vi "Panel.vi"(11 "ArrayHostPanel in":refnum<class "ArrayHostPanel.lvclass">) -> ()   [LabVIEW 2020, in "Nested.lvlib" / "ArrayHostPanel.lvclass"]
uses:
  ArrayHostPanel.lvclass
  C:/dev/lv/2020/lv-oopanel/OOPanel/Panel/Panel.lvclass
  OOPanel/Panel/Basic UI State.ctl
  ColorArrayPanel/ColorArrayPanel.lvclass
  C:/dev/lv/2020/lv-oopanel/OOPanel/ArrayPanel/ArrayPanel.lvclass
  OOPanel/ArrayManager/ArrayManager.lvclass
  OOPanel/Panel/Panel.lvclass
  OOPanel/OOPanel.lvlib
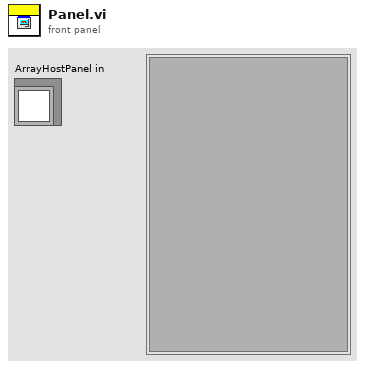
[diagram p1: front panel]
types:
  T1 = typedef "OOPanel.lvlib/Panel.lvclass/Basic UI State.ctl" = enum16{"Init", "Run", "Close"}
  T2 = typedef "OOPanel.lvlib/Panel.lvclass/Panel Events.ctl" = cluster{"Visbility":refnum<user-event>, "Close":refnum<user-event>}
  T3 = typedef "OOPanel.lvlib/Visibility State.ctl" = enum16{"Idle", "Closed", "Hidden", "Visible", "Subpanel", "Hidden Subpanel"}
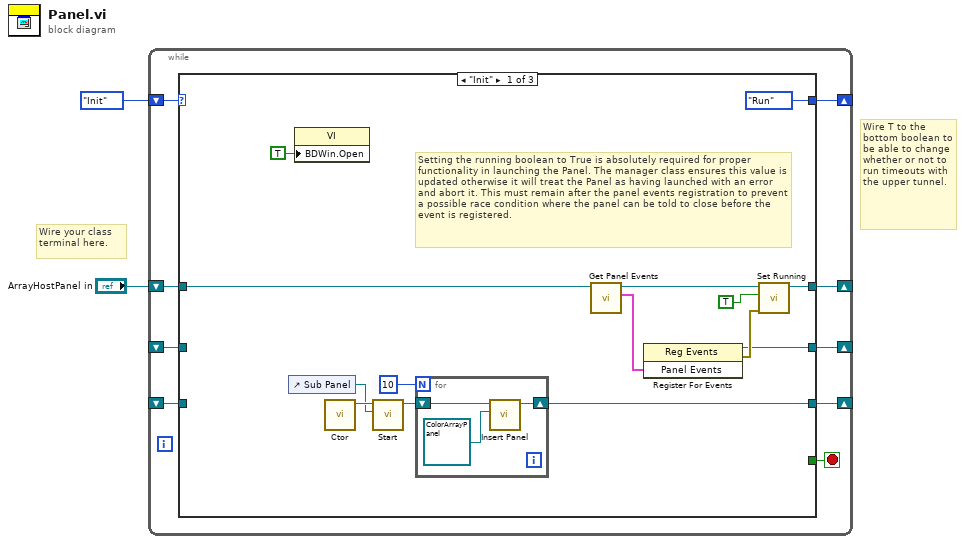
[diagram p0: block diagram]
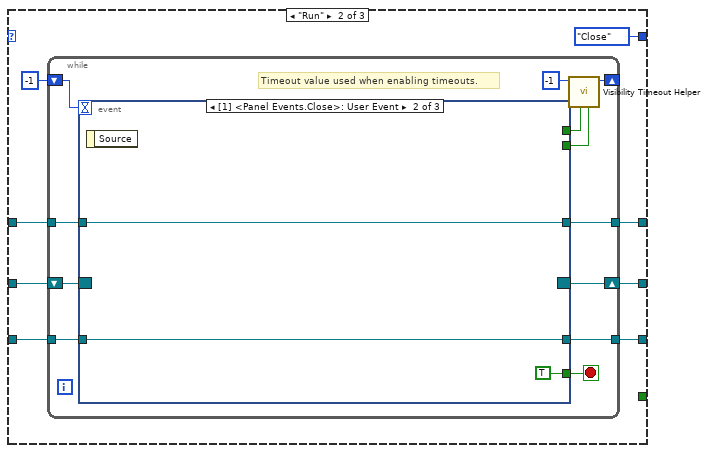
[diagram p2: hidden frame]
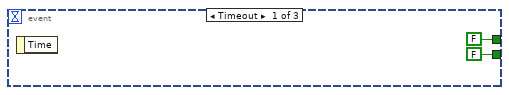
[diagram p3: hidden frame]
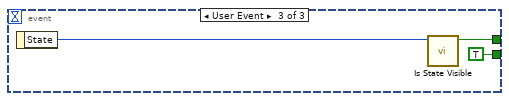
[diagram p4: hidden frame]
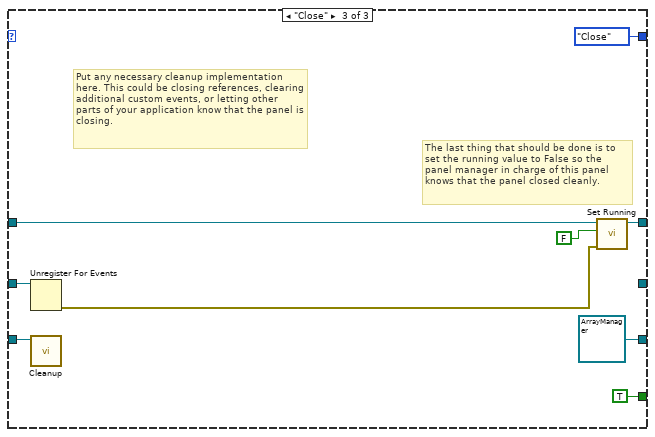
[diagram p5: hidden frame]
diagram:
  # "Wire T to the bottom boolean to be able to change whether or not to run timeouts with the upper tunnel."
  # "Wire your class terminal here."
  n1 = while {
    shift-right: [w10] -> _
    shift-left: _ -> [w11]
    shift-right: [w8] -> _
    shift-left: Basic_UI_State."Init" ("Basic UI State") -> [w9]
    shift-right: [w6] -> _
    shift-left: "ArrayHostPanel in" -> [w5]
    shift-right: [w4] -> _
    shift-left: _ -> [w3]
    stop <- w7 stop-if-true
    n2 = case shown="\"Init\"" w9 {
      tunnel: w11 -> [_ w36 w61]
      tunnel: [w22 w34 _] -> w10
      tunnel: [Basic_UI_State."Run" ("Basic UI State") Basic_UI_State."Close" ("Basic UI State") Basic_UI_State."Close" ("Basic UI State")] -> w8
      tunnel: [_ _ TRUE] -> w7
      tunnel: [w21 w31 w59] -> w6
      tunnel: w5 -> [w20 w32 w60]
      tunnel: [w13 w29 refnum<class "ArrayManager.lvclass"> refnum ("ArrayManager out")] -> w4
      tunnel: w3 -> [_ w30 w58]
      frame "Init" {
        # "Setting the running boolean to True is absolutely required for proper functionality in launching the Panel. The manager class ensures this value is updated otherwise it will treat the Panel as having launched with an error and abort it. This must remain after the panel events registration to prevent a possible race condition where the panel can be told to close before the event is registered."
        n3 = control-ref of="Sub Panel"() -> (w15:refnum<vi>)
        n4 = property class="VI"("BDWin.Open"=TRUE ("Block Diagram Window:Open")) -> ()  [unwired: 2 in, 2 out]
        n5 = call "Ctor.vi"() -> ("PanelArray"=w16:refnum<class "ArrayManager.lvclass">)  [unwired: 10 in, 1 out]
        n6 = call "Start.vi"("Container"=w15, "ArrayManager in"=w16) -> ("ArrayManager out"=w14:refnum<class "ArrayManager.lvclass">)  [unwired: 8 in, 1 out]
        n7 = for {
          N: 10 -> [_]
          shift-right: [w26] -> w13
          shift-left: w14 -> [w28]
          n8 = call "Insert Panel.vi"("Panel/Type"=refnum<class "ColorArrayPanel.lvclass"> refnum ("Nested.lvlib:ColorArrayPanel.lvclass"), "PanelArray in"=w28) -> ("PanelArray out"=w26:refnum<class "ArrayManager.lvclass">)  [unwired: 7 in, 2 out]
        }
        n9 = call "Get Panel Events.vi"("Panel in"=w20) -> ("Panel Events"=w18:T2, "Panel out"=w19:refnum<class "ArrayHostPanel.lvclass">)  [unwired: 8 in, 1 out]
        n10 = register-events(w18) -> (reference out=w22:refnum<event-registration>, error out=w24:errorcluster)  [unwired: 2 in]
        n11 = call "Set Running.vi"("error in (no error)"=w24, "Running"=TRUE, "Panel in"=w19) -> ("Panel out"=w21:refnum<class "ArrayHostPanel.lvclass">)  [unwired: 7 in, 1 out]
      }
      frame "Run" {
        n12 = while {
          shift-right: [w44] -> w34
          shift-left: w36 -> [w45]
          shift-right: [w47] -> _
          shift-left: -1 ("Timeout") -> [w46]
          tunnel: w32 -> [w40]
          tunnel: [w39] -> w31
          tunnel: w30 -> [w38]
          tunnel: [w37] -> w29
          stop <- w41 stop-if-true
          # "Timeout value used when enabling timeouts."
          n13 = event shown="[1] <Panel Events.Close>: User Event" {
            selector: w45 -> [_ _ _]
            dyn-events: [_ _ _] -> w44
            timeout: w46 -> [_ _ _]
            tunnel: [FALSE _ w55] -> w43
            tunnel: [FALSE _ TRUE] -> w42
            tunnel: [_ TRUE _] -> w41
            tunnel: w40 -> [_ w52 _]
            tunnel: [_ w52 _] -> w39
            tunnel: w38 -> [_ w51 _]
            tunnel: [_ w51 _] -> w37
            event Timeout {
              n14 = event-data() -> ()  [unwired: 1 in, 1 out]
            }
            event User Event {
              n15 = event-data() -> ()  [unwired: 1 in, 1 out]
            }
            event User Event {
              n16 = event-data() -> ("State"=w56:T3)  [unwired: 1 in]
              n17 = call "Is State Visible.vi"("Visibility"=w56) -> ("Visible"=w55:bool)  [unwired: 10 in]
            }
          }
          n18 = call "Visibility Timeout Helper.vi"("Update?"=w42, "Use Timeout?"=w43, "Visible Timeout mS"=-1) -> ("Timeout"=w47:i32)  [unwired: 8 in]
        }
      }
      frame "Close" {
        # "Put any necessary cleanup implementation here. This could be closing references, clearing additional custom events, or letting other parts of your application know that the panel is closing."
        # "The last thing that should be done is to set the running value to False so the panel manager in charge of this panel knows that the panel closed cleanly."
        n19 = Unregister For Events(event registration refnum=w61) -> (error out=w63:errorcluster)  [unwired: 1 in]
        n20 = call "Cleanup.vi"("PanelArray in"=w58) -> ()  [unwired: 10 in, 1 out]
        n21 = call "Set Running.vi"("error in (no error)"=w63, "Running"=FALSE, "Panel in"=w60) -> ("Panel out"=w59:refnum<class "ArrayHostPanel.lvclass">)  [unwired: 7 in, 1 out]
      }
    }
  }
